vi "Top Level FPGA_w8LED.vi"() -> ()   [LabVIEW 2012]
uses:
  <vilib>/Platform/TimedLoop/XDataNode/timing_clust.ctl
  <vilib>/Platform/TimedLoop/XDataNode/nitl_modes.ctl
  <vilib>/Platform/TimedLoop/XDataNode/wakeup.ctl
  <vilib>/rvi/DataTransferAndStorage/Container/Common/niFpgaContainerMetaDataKey.ctl
  <vilib>/rvi/DataTransferAndStorage/Container/Common/niFpgaContainerState.ctl
  <vilib>/rvi/DataTransferAndStorage/Container/Common/niFpgaDataTypeControl.ctl
  <vilib>/rvi/DataTransferAndStorage/Container/Common/niFpgaContainerImplementationControl.ctl
  <vilib>/rvi/DataTransferAndStorage/Container/Common/niFpgaContainerArbitrationOptionsControl.ctl
  <vilib>/rvi/DataTransferAndStorage/Container/Common/niFpgaTransferTypeControl.ctl
  <vilib>/rvi/DataTransferAndStorage/Container/Common/niFpgaContainerInitializationParameters.ctl
  <vilib>/rvi/Memory/Memory_Types/niFpgaMemoryInterfaceConfiguration.ctl
  <vilib>/rvi/FIFO/Fifo_Types/niFpgaFifoControlLogicControl.ctl
  <vilib>/rvi/eio/common/nirviEmuTemplateMethod_errors.vi
  <vilib>/rvi/FIFO/Fifo_Resource/nirvififoEmulationSetSize.vi
  <vilib>/rvi/DataTransferAndStorage/Container/Common/niFpgaContainerGetUniqueNameForEmu.vi
  <vilib>/rvi/Emulation/niFpgaSctlEmulationRegisterWithScheduler.vi
  <vilib>/rvi/Emulation/niFpgaSctlEmulationScheduler.vi
  <vilib>/rvi/DataTransferAndStorage/Container/Common/niFpgaContainerSetEmuInfo.vi
  <vilib>/rvi/eio/common/nirviEmuReportErrorAndStop.vi
  <vilib>/rvi/Emulation/niFpgaSctlEmulationFifoFullMgr.vi
  <vilib>/rvi/errors/niFpgaSetErrorForExecOnDevCompSimple.vi
  <vilib>/rvi/Memory/Memory_Emulation/nirvimemoryEmulationManagerCache_GetValue.vi
  <vilib>/rvi/Memory/Memory_Emulation/niFpgaMemoryEmulationValidateCache.vi
  <vilib>/rvi/Memory/Memory_Emulation/nirvimemoryEmulationManagerCache_InsertValue.vi
  <vilib>/rvi/Memory/Memory_Emulation/nirvimemoryEmulationManagerCache_SetValue.vi
  <vilib>/rvi/Emulation/niFpgaSctlEmulationResourceMgr.vi
  <vilib>/rvi/Memory/Memory_Emulation/niFpgaMemoryEmulationCacheClearOnFirstRun.vi
  <vilib>/rvi/Memory/Memory_Emulation/nirvimemoryEmulationManagerCache_MakeExclusive.vi
  <vilib>/rvi/Memory/Memory_Emulation/nirvimemoryEmulationManagerCache_ReleaseExclusive.vi
  <vilib>/Utility/error.llb/Clear Errors.vi
  <vilib>/eio/EIONode/EIONode.xnode
  <vilib>/Platform/TimedLoop/XDataNode/XDataNode.xnode
  <vilib>/rvi/DataTransferAndStorage/Container/XNode/niFpgaContainer.xnode
  <vilib>/rvi/FIFO/Fifo_Resource/nirvififoEmulationClear.vi
  <vilib>/rvi/LocalResourceManager/LocalResourceManager.xnode
  <vilib>/rvi/FIFO/Fifo_Resource/nirvififoEmulationRead.vi
  <vilib>/rvi/DataTransferAndStorage/Register/Emulation/niFpgaRegisterEmulation.vi
  <vilib>/rvi/Memory/Memory_Emulation/nirvimemoryEmulation.vi
  <vilib>/rvi/FIFO/Fifo_Resource/nirvififoEmulationWrite.vi
  <vilib>/Platform/TimedLoop/XDataNode/XDNodeRunTimeDep.lvlib
panel:
  in  "Testpulse separation (20 ns ticks)":u32=50000
  in  "channel 7 on/off":bool
  in  "channel 6 on/off":bool
  in  "channel 5 on/off":bool
  in  "channel 4 on/off":bool
  in  "channel 3 on/off":bool
  in  "channel 1 on/off":bool
  in  "channel 2 on/off":bool
  in  "channel 0 on/off":bool
  out "Timestamp":u64
  in  "Stop FPGA and exit":bool
  out "DMA FIFO Timed Out?":bool
  in  "Testpulser On/Off":bool
  in  "Testpulse Time Delay (20 ns ticks)":u32=15
  in  "Testpulse duration (20 ns ticks)":u32=1
  in  "location":i16(ring) items=["Purdue", "NIKHEF", "Zurich", "???"]
  in  "initial value":u64
  in  "circular buffer length":u32=1000
  in  "# of pretrigger":u32=20
  out "IO Module\\Pll Unlocked":bool
  out "IO Module\\ADC Error B":bool
  out "IO Module\\ADC Error A":bool
  out "Init Done":bool
  in  "Trigger 4":i16=4000
  in  "Trigger 5":i16=4000
  in  "Trigger 6":i16=4000
  in  "Trigger 7":i16=4000
  in  "Trigger 2":i16=4000
  in  "Trigger 3":i16=4000
  in  "Trigger 1":i16=4000
  in  "Record Size only data":u32=95
  in  "Trigger 0":i16=4000
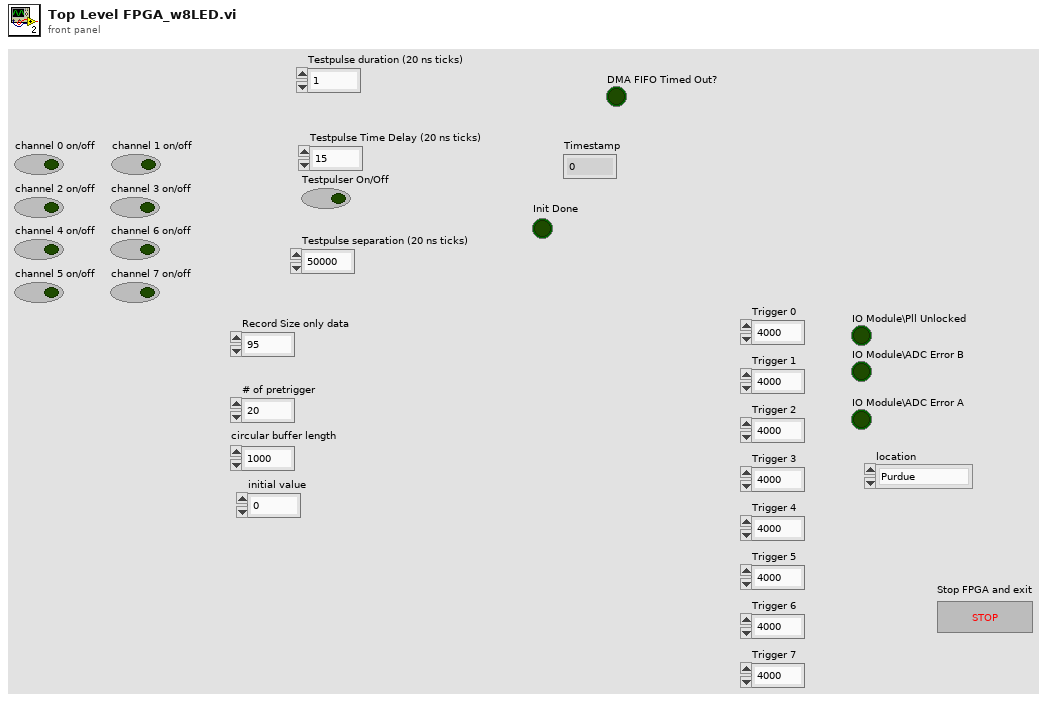
[diagram p1: front panel]
types:
  T1 = typedef "XDNodeRunTimeDep.lvlib/timing_clust.ctl" = cluster{"Expected End [f-1]":u64, "Actual End [f-1]":u64, "Finished Late? [f-1]":bool, "Expected End [i-1]":u64, "Actual End [i-1]":u64, "Finished Late? [i-1]":bool, "Expected Start [i]":u64, "Actual Start [i]":u64, "Expected Start [f]":u64, "Actual Start [f]":u64, "Source Name":string, "Structure Name":string, "Period":i64, "Deadline":i64, "Offset":i64, "Start":i64, "Priority":i32, "Timeout":i32, "Mode":T2, "Wakeup Reason":T3, "Error":errorcluster, "Source Type":string, "Secondary Source Type":string, "Global End Time":u64, "Global Start Time":u64, "Frame Duration":u64, "Iteration Duration":u64, "Assigned CPU":i32, "I/O Scan Engine Mode":u32}
  T2 = typedef "XDNodeRunTimeDep.lvlib/nitl_modes.ctl" = enum32{"No Change", "Process missed periods, maintain original phase", "Discard missed periods, maintain original phase", "Process missed periods, ignore original phase", "Discard missed periods, ignore original phase"}
  T3 = typedef "XDNodeRunTimeDep.lvlib/wakeup.ctl" = enum32{"Normal", "Aborted", "Asynchronous wakeup", "Timing source error", "Timed loop error", "Timeout"}
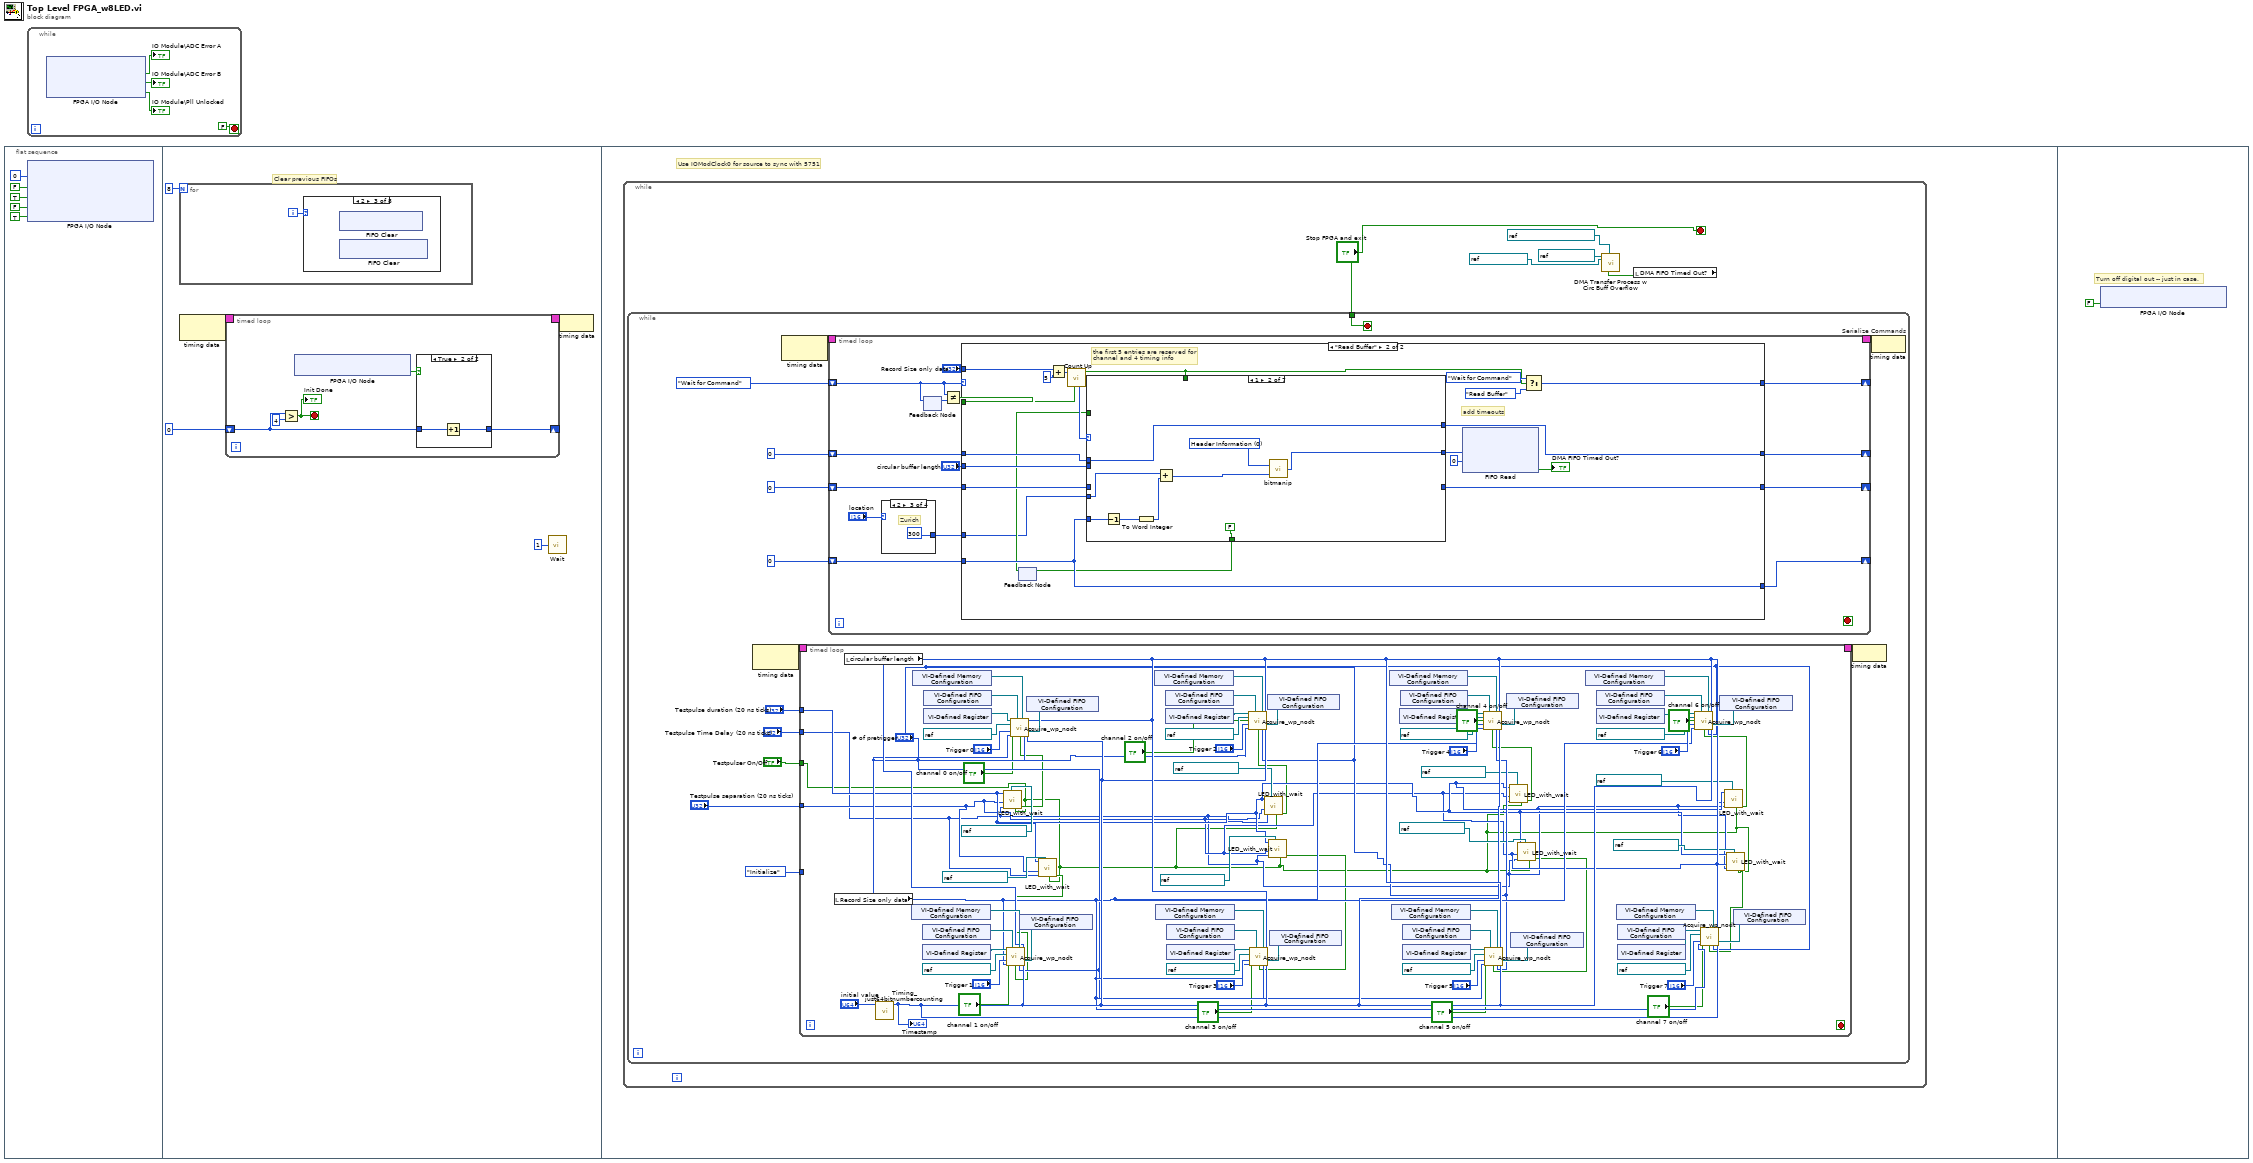
[diagram p0: block diagram]
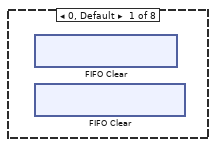
[diagram p2: hidden frame]
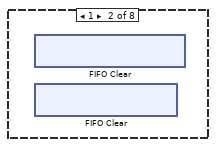
[diagram p3: hidden frame]
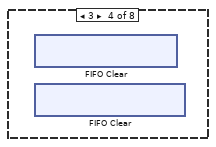
[diagram p4: hidden frame]
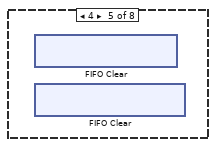
[diagram p5: hidden frame]
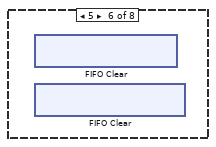
[diagram p6: hidden frame]
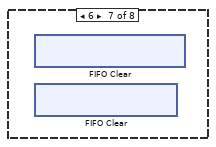
[diagram p7: hidden frame]
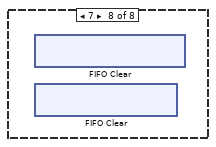
[diagram p8: hidden frame]
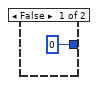
[diagram p9: hidden frame]
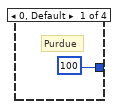
[diagram p10: hidden frame]
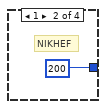
[diagram p11: hidden frame]
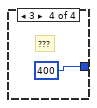
[diagram p12: hidden frame]
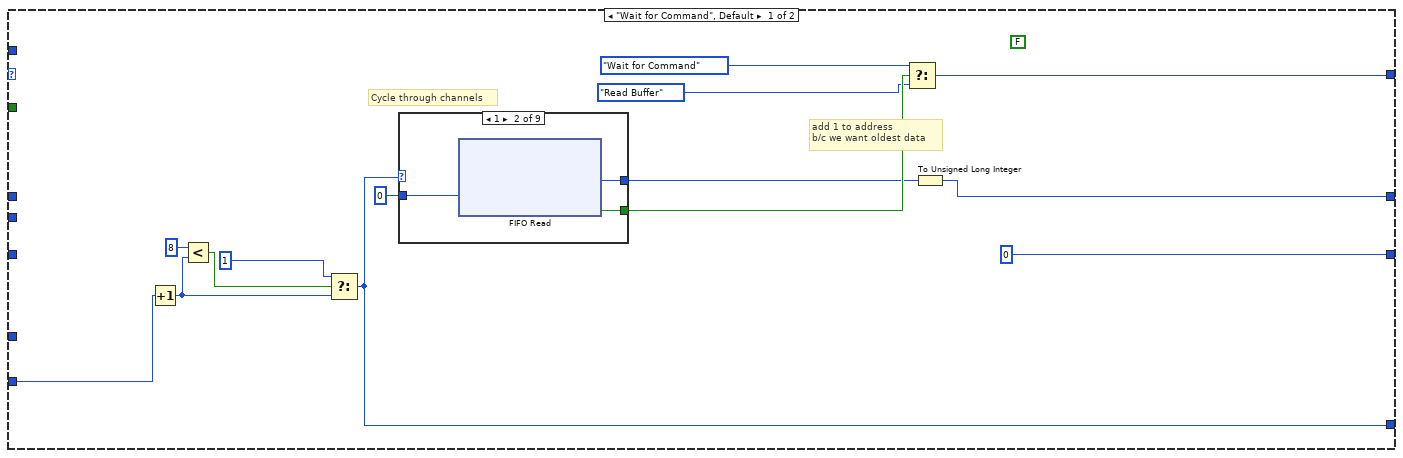
[diagram p13: hidden frame]
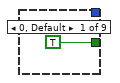
[diagram p14: hidden frame]
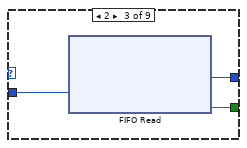
[diagram p15: hidden frame]
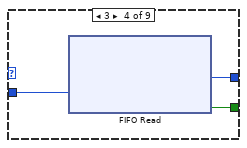
[diagram p16: hidden frame]
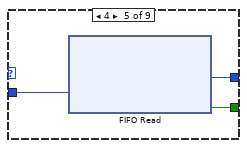
[diagram p17: hidden frame]
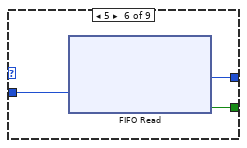
[diagram p18: hidden frame]
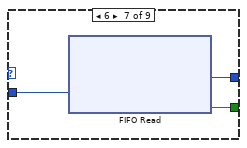
[diagram p19: hidden frame]
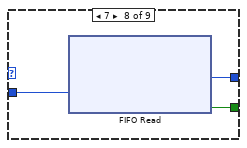
[diagram p20: hidden frame]
diagram:
  n1 = flat-sequence {
    frame #0 {
      n2 = xnode "FPGA I/O Node"("IO Module\\Sample Clock Select"=u8 0 ("IO Module\\Sample Clock Select"), "IO Module\\Force Initialization"=FALSE ("IO Module\\Force Initialization"), "IO Module\\Force Initialization"=TRUE ("IO Module\\Force Initialization"), "IO Module\\Force Initialization"=FALSE ("IO Module\\Force Initialization"), "IO Module\\Digital Output Enable"=TRUE ("IO Module\\Digital Output Enable")) -> ()  [unwired: 5 in, 5 out]
    }
    frame #1 {
      # "Clear previous FIFOs"
      n3 = for {
        N: 8 -> [_]
        i -> [w11]
        n4 = case shown="2" w11 {
          frame 0, Default {
            n5 = xnode ("FIFO Clear")() -> ()  [unwired: 1 in, 1 out]
            n6 = xnode ("FIFO Clear")() -> ()  [unwired: 1 in, 1 out]
          }
          frame 1 {
            n7 = xnode ("FIFO Clear")() -> ()  [unwired: 1 in, 1 out]
            n8 = xnode ("FIFO Clear")() -> ()  [unwired: 1 in, 1 out]
          }
          frame 2 {
            n9 = xnode ("FIFO Clear")() -> ()  [unwired: 1 in, 1 out]
            n10 = xnode ("FIFO Clear")() -> ()  [unwired: 1 in, 1 out]
          }
          frame 3 {
            n11 = xnode ("FIFO Clear")() -> ()  [unwired: 1 in, 1 out]
            n12 = xnode ("FIFO Clear")() -> ()  [unwired: 1 in, 1 out]
          }
          frame 4 {
            n13 = xnode ("FIFO Clear")() -> ()  [unwired: 1 in, 1 out]
            n14 = xnode ("FIFO Clear")() -> ()  [unwired: 1 in, 1 out]
          }
          frame 5 {
            n15 = xnode ("FIFO Clear")() -> ()  [unwired: 1 in, 1 out]
            n16 = xnode ("FIFO Clear")() -> ()  [unwired: 1 in, 1 out]
          }
          frame 6 {
            n17 = xnode ("FIFO Clear")() -> ()  [unwired: 1 in, 1 out]
            n18 = xnode ("FIFO Clear")() -> ()  [unwired: 1 in, 1 out]
          }
          frame 7 {
            n19 = xnode ("FIFO Clear")() -> ()  [unwired: 1 in, 1 out]
            n20 = xnode ("FIFO Clear")() -> ()  [unwired: 1 in, 1 out]
          }
        }
      }
      n21 = node-c288() -> (w10:T1)  [unwired: 1 in]
      n22 = timed-loop {
        shift-right: [w15] -> _
        shift-left: u16 0 -> [w14]
        timing: w10 -> [_]
        timing-out: [_] -> w9
        stop <- w12 stop-if-true
        n23 = Greater?(x=w14, y=u16 4) -> (0:w12:bool)
        "Init Done" <- w12
        n24 = xnode "FPGA I/O Node"() -> ("IO Module\\Initialization Done"=w16:bool)  [unwired: 1 in, 1 out]
        n25 = case shown="True" w16 {
          tunnel: [u16 0 w19] -> w15
          tunnel: w14 -> [_ w18]
          frame False {
          }
          frame True {
            n26 = Increment(x=w18) -> (x+1=w19:u16)
          }
        }
      }
      n27 = call "Wait"("Count(mSec)"=u32 1) -> ()  [unwired: 1 out]
      n28 = node-c288(w9) -> ()
    }
    frame #2 {
      # "Use IOModClock0 for source to sync with 5751"
      n29 = while {
        stop <- "Stop FPGA and exit" stop-if-true
        n30 = while {
          tunnel: "Stop FPGA and exit" -> [w34]
          stop <- w34 stop-if-true
          n31 = node-c288() -> (w40:T1)  [unwired: 1 in]
          n32 = node-c288() -> (w42:T1)  [unwired: 1 in]
          n33 = timed-loop {
            timing: w40 -> [_]
            timing-out: [_] -> w39
            tunnel: "Testpulser On/Off" -> [w43]
            tunnel: "Testpulse Time Delay (20 ns ticks)" -> [w50]
            tunnel: "Testpulse duration (20 ns ticks)" -> [w52]
            tunnel: enum16{"Initialize", "Get New Value", "Wait"}."Initialize" ("State In") -> [_]
            tunnel: "Testpulse separation (20 ns ticks)" -> [w51]
            stop <- _ stop-if-true
            n34 = local read "Record Size only data"() -> (w73:u32)
            n35 = local read "circular buffer length"() -> (w75:u32)
            n36 = call "Timing_just64bitnumbercounting.vi"("initial value"="initial value") -> ("x+1"=w74:u64)  [unwired: 10 in]
            "Timestamp" <- w74
            n37 = xnode "VI-Defined Memory Configuration"() -> ("Memory Out"=w122:refnum<k21>)
            n38 = xnode "VI-Defined Memory Configuration"() -> ("Memory Out"=w76:refnum<k21>)
            n39 = xnode "VI-Defined FIFO Configuration"() -> ("FIFO Out"=w121:refnum<k21>)
            n40 = xnode "VI-Defined Register"() -> ("Register Out"=w102:refnum<k21>)
            n41 = xnode "VI-Defined FIFO Configuration"() -> ("FIFO Out"=w77:refnum<k21>)
            n42 = xnode "VI-Defined Register"() -> ("Register Out"=w72:refnum<k21>)
            n43 = call "LED_with_wait.vi"("Testpulser On/Off"=w43, "FPGA I/O In"=refnum<k21> "IO Module\\D0 0", "Testpulse Time Delay (20 ns ticks)"=w50, "Testpulse Separation (20 ns ticks)"=w51, "Testpulse duration (20 ns ticks)"=w52) -> ("Is Test Pulse?"=w61:bool)  [unwired: 5 in, 1 out]
            n44 = xnode "VI-Defined FIFO Configuration"() -> ("FIFO Out"=w88:refnum<k21>)
            n45 = xnode "VI-Defined FIFO Configuration"() -> ("FIFO Out"=w80:refnum<k21>)
            n46 = call "Acquire_wp_nodt.vi"("Ch Armed Reg"=w72, "Command FIFO"=w77, "Circular Buffer Mem"=w76, "circular buffer length"=w75, "FPGA I/O In"=refnum<k21> "IO Module\\AI A0", "channel on/off"="channel 0 on/off", "Trigger"="Trigger 0", "Timing FIFO"=w80, "Samples to Acquire"=w73, "Is Test Pulse?"=w61, "# of pretrigger"="# of pretrigger", "timing"=w74) -> ()  [unwired: 4 in]
            n47 = call "LED_with_wait.vi"("Testpulser On/Off"=w43, "FPGA I/O In"=refnum<k21> "IO Module\\D0 1", "Testpulse Time Delay (20 ns ticks)"=w50, "Testpulse Separation (20 ns ticks)"=w51, "Testpulse duration (20 ns ticks)"=w52) -> ("Is Test Pulse?"=w60:bool)  [unwired: 5 in, 1 out]
            n48 = call "Acquire_wp_nodt.vi"("Ch Armed Reg"=w102, "Command FIFO"=w121, "Circular Buffer Mem"=w122, "circular buffer length"=w75, "FPGA I/O In"=refnum<k21> "IO Module\\AI A1", "channel on/off"="channel 1 on/off", "Trigger"="Trigger 1", "Timing FIFO"=w88, "Samples to Acquire"=w73, "Is Test Pulse?"=w60, "# of pretrigger"="# of pretrigger", "timing"=w74) -> ()  [unwired: 4 in]
            n49 = xnode "VI-Defined Memory Configuration"() -> ("Memory Out"=w116:refnum<k21>)
            n50 = xnode "VI-Defined Memory Configuration"() -> ("Memory Out"=w119:refnum<k21>)
            n51 = xnode "VI-Defined FIFO Configuration"() -> ("FIFO Out"=w115:refnum<k21>)
            n52 = xnode "VI-Defined Register"() -> ("Register Out"=w98:refnum<k21>)
            n53 = xnode "VI-Defined FIFO Configuration"() -> ("FIFO Out"=w120:refnum<k21>)
            n54 = xnode "VI-Defined Register"() -> ("Register Out"=w100:refnum<k21>)
            n55 = call "LED_with_wait.vi"("Testpulser On/Off"=w43, "FPGA I/O In"=refnum<k21> "IO Module\\D0 2", "Testpulse Time Delay (20 ns ticks)"=w50, "Testpulse Separation (20 ns ticks)"=w51, "Testpulse duration (20 ns ticks)"=w52) -> ("Is Test Pulse?"=w45:bool)  [unwired: 5 in, 1 out]
            n56 = xnode "VI-Defined FIFO Configuration"() -> ("FIFO Out"=w87:refnum<k21>)
            n57 = call "Acquire_wp_nodt.vi"("Ch Armed Reg"=w98, "Command FIFO"=w115, "Circular Buffer Mem"=w116, "circular buffer length"=w75, "FPGA I/O In"=refnum<k21> "IO Module\\AI A2", "channel on/off"="channel 2 on/off", "Trigger"="Trigger 2", "Timing FIFO"=w87, "Samples to Acquire"=w73, "Is Test Pulse?"=w45, "# of pretrigger"="# of pretrigger", "timing"=w74) -> ()  [unwired: 4 in]
            n58 = call "LED_with_wait.vi"("Testpulser On/Off"=w43, "FPGA I/O In"=refnum<k21> "IO Module\\D0 3", "Testpulse Time Delay (20 ns ticks)"=w50, "Testpulse Separation (20 ns ticks)"=w51, "Testpulse duration (20 ns ticks)"=w52) -> ("Is Test Pulse?"=w44:bool)  [unwired: 5 in, 1 out]
            n59 = xnode "VI-Defined FIFO Configuration"() -> ("FIFO Out"=w86:refnum<k21>)
            n60 = call "Acquire_wp_nodt.vi"("Ch Armed Reg"=w100, "Command FIFO"=w120, "Circular Buffer Mem"=w119, "circular buffer length"=w75, "FPGA I/O In"=refnum<k21> "IO Module\\AI A3", "channel on/off"="channel 3 on/off", "Trigger"="Trigger 3", "Timing FIFO"=w86, "Samples to Acquire"=w73, "Is Test Pulse?"=w44, "# of pretrigger"="# of pretrigger", "timing"=w74) -> ()  [unwired: 4 in]
            n61 = xnode "VI-Defined Memory Configuration"() -> ("Memory Out"=w104:refnum<k21>)
            n62 = xnode "VI-Defined Memory Configuration"() -> ("Memory Out"=w107:refnum<k21>)
            n63 = xnode "VI-Defined Register"() -> ("Register Out"=w92:refnum<k21>)
            n64 = xnode "VI-Defined FIFO Configuration"() -> ("FIFO Out"=w103:refnum<k21>)
            n65 = xnode "VI-Defined FIFO Configuration"() -> ("FIFO Out"=w108:refnum<k21>)
            n66 = xnode "VI-Defined Register"() -> ("Register Out"=w96:refnum<k21>)
            n67 = xnode "VI-Defined FIFO Configuration"() -> ("FIFO Out"=w85:refnum<k21>)
            n68 = call "LED_with_wait.vi"("Testpulser On/Off"=w43, "FPGA I/O In"=refnum<k21> "IO Module\\D0 4", "Testpulse Time Delay (20 ns ticks)"=w50, "Testpulse Separation (20 ns ticks)"=w51, "Testpulse duration (20 ns ticks)"=w52) -> ("Is Test Pulse?"=w46:bool)  [unwired: 5 in, 1 out]
            n69 = call "Acquire_wp_nodt.vi"("Ch Armed Reg"=w92, "Command FIFO"=w103, "Circular Buffer Mem"=w104, "circular buffer length"=w75, "FPGA I/O In"=refnum<k21> "IO Module\\AI A4", "channel on/off"="channel 4 on/off", "Trigger"="Trigger 4", "Timing FIFO"=w85, "Samples to Acquire"=w73, "Is Test Pulse?"=w46, "# of pretrigger"="# of pretrigger", "timing"=w74) -> ()  [unwired: 4 in]
            n70 = xnode "VI-Defined FIFO Configuration"() -> ("FIFO Out"=w84:refnum<k21>)
            n71 = call "LED_with_wait.vi"("Testpulser On/Off"=w43, "FPGA I/O In"=refnum<k21> "IO Module\\D0 5", "Testpulse Time Delay (20 ns ticks)"=w50, "Testpulse Separation (20 ns ticks)"=w51, "Testpulse duration (20 ns ticks)"=w52) -> ("Is Test Pulse?"=w47:bool)  [unwired: 5 in, 1 out]
            n72 = call "Acquire_wp_nodt.vi"("Ch Armed Reg"=w96, "Command FIFO"=w108, "Circular Buffer Mem"=w107, "circular buffer length"=w75, "FPGA I/O In"=refnum<k21> "IO Module\\AI A5", "channel on/off"="channel 5 on/off", "Trigger"="Trigger 5", "Timing FIFO"=w84, "Samples to Acquire"=w73, "Is Test Pulse?"=w47, "# of pretrigger"="# of pretrigger", "timing"=w74) -> ()  [unwired: 4 in]
            n73 = xnode "VI-Defined Memory Configuration"() -> ("Memory Out"=w113:refnum<k21>)
            n74 = xnode "VI-Defined FIFO Configuration"() -> ("FIFO Out"=w114:refnum<k21>)
            n75 = xnode "VI-Defined Register"() -> ("Register Out"=w94:refnum<k21>)
            n76 = xnode "VI-Defined Memory Configuration"() -> ("Memory Out"=w110:refnum<k21>)
            n77 = xnode "VI-Defined FIFO Configuration"() -> ("FIFO Out"=w109:refnum<k21>)
            n78 = xnode "VI-Defined Register"() -> ("Register Out"=w90:refnum<k21>)
            n79 = xnode "VI-Defined FIFO Configuration"() -> ("FIFO Out"=w83:refnum<k21>)
            n80 = call "LED_with_wait.vi"("Testpulser On/Off"=w43, "FPGA I/O In"=refnum<k21> "IO Module\\D0 6", "Testpulse Time Delay (20 ns ticks)"=w50, "Testpulse Separation (20 ns ticks)"=w51, "Testpulse duration (20 ns ticks)"=w52) -> ("Is Test Pulse?"=w48:bool)  [unwired: 5 in, 1 out]
            n81 = call "Acquire_wp_nodt.vi"("Ch Armed Reg"=w94, "Command FIFO"=w114, "Circular Buffer Mem"=w113, "circular buffer length"=w75, "FPGA I/O In"=refnum<k21> "IO Module\\AI A6", "channel on/off"="channel 6 on/off", "Trigger"="Trigger 6", "Timing FIFO"=w83, "Samples to Acquire"=w73, "Is Test Pulse?"=w48, "# of pretrigger"="# of pretrigger", "timing"=w74) -> ()  [unwired: 4 in]
            n82 = call "LED_with_wait.vi"("Testpulser On/Off"=w43, "FPGA I/O In"=refnum<k21> "IO Module\\D0 7", "Testpulse Time Delay (20 ns ticks)"=w50, "Testpulse Separation (20 ns ticks)"=w51, "Testpulse duration (20 ns ticks)"=w52) -> ("Is Test Pulse?"=w49:bool)  [unwired: 5 in, 1 out]
            n83 = xnode "VI-Defined FIFO Configuration"() -> ("FIFO Out"=w82:refnum<k21>)
            n84 = call "Acquire_wp_nodt.vi"("Ch Armed Reg"=w90, "Command FIFO"=w109, "Circular Buffer Mem"=w110, "circular buffer length"=w75, "FPGA I/O In"=refnum<k21> "IO Module\\AI A7", "channel on/off"="channel 7 on/off", "Trigger"="Trigger 7", "Timing FIFO"=w82, "Samples to Acquire"=w73, "Is Test Pulse?"=w49, "# of pretrigger"="# of pretrigger", "timing"=w74) -> ()  [unwired: 4 in]
          }
          n85 = timed-loop "Serialize Commands" {
            timing: w42 -> [_]
            timing-out: [_] -> w41
            shift-right: [w904] -> _
            shift-left: enum16{"Wait for Command", "Read Buffer"}."Wait for Command" -> [w902]
            shift-right: [w908] -> _
            shift-left: u32 0 ("Element") -> [w907]
            shift-right: [w906] -> _
            shift-left: u8 0 ("t") -> [w905]
            shift-right: [w899] -> _
            shift-left: u64 0 ("Element") -> [w898]
            stop <- _ stop-if-true
            n86 = case shown="2" "location" {
              tunnel: [i16 100 i16 200 i16 300 i16 400] -> w896
              frame 0, Default {
                # "Purdue"
              }
              frame 1 {
                # "NIKHEF"
              }
              frame 2 {
                # "Zurich"
              }
              frame 3 {
                # "???"
              }
            }
            n87 = feedback-in #1(w902) -> ()
            n88 = feedback #1() -> (w903:enum16{"Wait for Command", "Read Buffer"})  [unwired: 1 in]
            n89 = Not Equal?(x=w902, y=w903) -> (x != y?=w900:bool)
            n90 = case shown="\"Read Buffer\"" w902 {
              tunnel: "Record Size only data" -> [_ w962]
              tunnel: [w916 w972] -> w906
              tunnel: w905 -> [w918 w972]
              tunnel: [w919 w957] -> w908
              tunnel: w907 -> [_ w971]
              tunnel: [w922 w973] -> w904
              tunnel: "circular buffer length" -> [_ w970]
              tunnel: w900 -> [_ w964]
              tunnel: [u64 0 ("Element") w959] -> w899
              tunnel: w898 -> [_ w958]
              tunnel: w896 -> [_ w953]
              frame "Wait for Command", Default {
                (unwired) FALSE
                # "add 1 to address\nb/c we want oldest data"
                # "Cycle through channels"
                n91 = Increment(x=w918) -> (x+1=w917:u8)
                n92 = Less?(x=u8 8, y=w917) -> (x < y?=w926:bool)
                n93 = Select(t=u8 1, s=w926, f=w917) -> (s? t:f=w916:u8)
                n94 = case shown="1" w916 {
                  tunnel: [TRUE ("Timed Out?") w931 w932 w935 w938 w941 w944 w947 w950] -> w923
                  tunnel: 0 ("Timeout") -> [_ w930 w934 w937 w940 w943 w946 w949 w952]
                  tunnel: [_ w929 w933 w936 w939 w942 w945 w948 w951] -> w915
                  frame 0, Default {
                  }
                  frame 1 {
                    n95 = xnode ("FIFO Read")("Timeout"=w930) -> ("Element"=w929:i16, "Timed Out?"=w931:bool)  [unwired: 1 in, 1 out]
                  }
                  frame 2 {
                    n96 = xnode ("FIFO Read")("Timeout"=w934) -> ("Element"=w933:i16, "Timed Out?"=w932:bool)  [unwired: 1 in, 1 out]
                  }
                  frame 3 {
                    n97 = xnode ("FIFO Read")("Timeout"=w937) -> ("Element"=w936:i16, "Timed Out?"=w935:bool)  [unwired: 1 in, 1 out]
                  }
                  frame 4 {
                    n98 = xnode ("FIFO Read")("Timeout"=w940) -> ("Element"=w939:i16, "Timed Out?"=w938:bool)  [unwired: 1 in, 1 out]
                  }
                  frame 5 {
                    n99 = xnode ("FIFO Read")("Timeout"=w943) -> ("Element"=w942:i16, "Timed Out?"=w941:bool)  [unwired: 1 in, 1 out]
                  }
                  frame 6 {
                    n100 = xnode ("FIFO Read")("Timeout"=w946) -> ("Element"=w945:i16, "Timed Out?"=w944:bool)  [unwired: 1 in, 1 out]
                  }
                  frame 7 {
                    n101 = xnode ("FIFO Read")("Timeout"=w949) -> ("Element"=w948:i16, "Timed Out?"=w947:bool)  [unwired: 1 in, 1 out]
                  }
                  frame 8 {
                    n102 = xnode ("FIFO Read")("Timeout"=w952) -> ("Element"=w951:i16, "Timed Out?"=w950:bool)  [unwired: 1 in, 1 out]
                  }
                }
                n103 = Select(t=enum16{"Wait for Command", "Read Buffer"}."Wait for Command", s=w923, f=enum16{"Wait for Command", "Read Buffer"}."Read Buffer") -> (s? t:f=w922:enum16{"Wait for Command", "Read Buffer"})
                n104 = To Unsigned Long Integer(number=w915) -> (unsigned 32bit integer=w919:u32)
              }
              frame "Read Buffer" {
                # "the first 5 entries are reserved for channel and 4 timing info"
                # "add timeouts"
                n105 = feedback #2() -> (w956:bool)  [unwired: 1 in]
                n106 = Add(x=w962, y=u32 5) -> (x+y=w960:u32)
                n107 = call "Count Up.vi"("Reset?"=w964, "goal"=w960) -> ("Count Met"=w966:bool, "count"=w963:u32)  [unwired: 8 in]
                n108 = case shown="1" w963 {
                  tunnel: w972 -> [_ w980 w989 _ _ _ w1028]
                  tunnel: w971 -> [_ w986 w991 w1012 w1018 w1024 w1035]
                  tunnel: w970 -> [_ _ _ _ _ _ w1034]
                  tunnel: w966 -> [_ _ _ _ _ _ w1033]
                  tunnel: [i16 0 ("Data") w983 w993 w1010 w1016 w1022 w1029] -> w965
                  tunnel: w956 -> [_ _ _ _ _ _ w1031]
                  tunnel: [u64 0 ("Element") _ w990 w1013 w1019 w1025 _] -> w959
                  tunnel: w958 -> [_ _ _ w1013 w1019 w1025 _]
                  tunnel: [u32 0 ("Element") w986 w991 w1012 w1018 w1024 _] -> w957
                  tunnel: [FALSE FALSE FALSE FALSE FALSE TRUE FALSE] -> w955
                  tunnel: w953 -> [_ w978 _ _ _ _ _]
                  frame 0, Default {
                  }
                  frame 1 {
                    w982 = u16 0 items=["Header Information", "Particle Pulse", "Test Pulse"] ("Pulse Type")
                    n109 = Decrement(x=w980) -> (x-1=w981:u8)
                    n110 = To Word Integer(number=w981) -> (16bit integer=w979:i16)
                    n111 = Add(x=w978, y=w979) -> (x+y=w984:i16)
                    n112 = call "bitmanip.vi"("Pulse Type"=w982, "Integer to be written"=w984) -> ("Integer Written"=w983:i16)  [unwired: 2 in]
                  }
                  frame 2 {
                    # "reads out the lsb of the timing information"
                    n113 = case shown="2" w989 {
                      tunnel: [_ w994 w996 w998 w1000 w1002 w1004 w1006 w1008] -> w990
                      frame Default {
                      }
                      frame 1 {
                        n114 = xnode ("FIFO Read")("Timeout"=0) -> ("Element"=w994:u64)  [unwired: 1 in, 2 out]
                      }
                      frame 2 {
                        n115 = xnode ("FIFO Read")("Timeout"=0) -> ("Element"=w996:u64)  [unwired: 1 in, 2 out]
                      }
                      frame 3 {
                        n116 = xnode ("FIFO Read")("Timeout"=0) -> ("Element"=w998:u64)  [unwired: 1 in, 2 out]
                      }
                      frame 4 {
                        n117 = xnode ("FIFO Read")("Timeout"=0) -> ("Element"=w1000:u64)  [unwired: 1 in, 2 out]
                      }
                      frame 5 {
                        n118 = xnode ("FIFO Read")("Timeout"=0) -> ("Element"=w1002:u64)  [unwired: 1 in, 2 out]
                      }
                      frame 6 {
                        n119 = xnode ("FIFO Read")("Timeout"=0) -> ("Element"=w1004:u64)  [unwired: 1 in, 2 out]
                      }
                      frame 7 {
                        n120 = xnode ("FIFO Read")("Timeout"=0) -> ("Element"=w1006:u64)  [unwired: 1 in, 2 out]
                      }
                      frame 8 {
                        n121 = xnode ("FIFO Read")("Timeout"=0) -> ("Element"=w1008:u64)  [unwired: 1 in, 2 out]
                      }
                    }
                    n122 = Split Number(x=w990) -> (hi(x)=w988:u32)  [unwired: 1 out]
                    n123 = Split Number(x=w988) -> (hi(x)=w987:u16)  [unwired: 1 out]
                    n124 = To Word Integer(number=w987) -> (16bit integer=w993:i16)
                  }
                  frame 3 {
                    n125 = Split Number(x=w1013) -> (hi(x)=w1015:u32)  [unwired: 1 out]
                    n126 = Split Number(x=w1015) -> (lo(x)=w1014:u16)  [unwired: 1 out]
                    n127 = To Word Integer(number=w1014) -> (16bit integer=w1010:i16)
                  }
                  frame 4 {
                    n128 = Split Number(x=w1019) -> (lo(x)=w1021:u32)  [unwired: 1 out]
                    n129 = Split Number(x=w1021) -> (hi(x)=w1020:u16)  [unwired: 1 out]
                    n130 = To Word Integer(number=w1020) -> (16bit integer=w1016:i16)
                  }
                  frame 5 {
                    n131 = Split Number(x=w1025) -> (lo(x)=w1027:u32)  [unwired: 1 out]
                    n132 = Split Number(x=w1027) -> (lo(x)=w1026:u16)  [unwired: 1 out]
                    n133 = To Word Integer(number=w1026) -> (16bit integer=w1022:i16)
                  }
                  frame 6.. {
                    n134 = call "Circular Buffer Address_try_without_deadtime.vi"("Reset?"=w1031, "Starting Address"=w1035, "circular buffer length"=w1034) -> ("Address"=w1032:u32)  [unwired: 8 in]
                    n135 = case shown="1" w1028 {
                      tunnel: w1032 -> [_ w1039 w1042 w1045 w1048 w1051 w1054 w1057 w1060]
                      tunnel: w1033 -> [_ w1038 w1041 w1044 w1047 w1050 w1053 w1056 w1059]
                      tunnel: [i16 0 w1037 w1040 w1043 w1046 w1049 w1052 w1055 w1058] -> w1029
                      frame Default {
                        # "Error"
                      }
                      frame 1 {
                        n136 = xnode ("Memory Read")("Address"=w1039) -> ("Data"=w1037:i16)  [unwired: 1 in, 1 out]
                        n137 = xnode ("Register Write")("Data"=w1038) -> ()  [unwired: 1 in, 1 out]
                      }
                      frame 2 {
                        n138 = xnode ("Memory Read")("Address"=w1042) -> ("Data"=w1040:i16)  [unwired: 1 in, 1 out]
                        n139 = xnode ("Register Write")("Data"=w1041) -> ()  [unwired: 1 in, 1 out]
                      }
                      frame 3 {
                        n140 = xnode ("Memory Read")("Address"=w1045) -> ("Data"=w1043:i16)  [unwired: 1 in, 1 out]
                        n141 = xnode ("Register Write")("Data"=w1044) -> ()  [unwired: 1 in, 1 out]
                      }
                      frame 4 {
                        n142 = xnode ("Memory Read")("Address"=w1048) -> ("Data"=w1046:i16)  [unwired: 1 in, 1 out]
                        n143 = xnode ("Register Write")("Data"=w1047) -> ()  [unwired: 1 in, 1 out]
                      }
                      frame 5 {
                        n144 = xnode ("Memory Read")("Address"=w1051) -> ("Data"=w1049:i16)  [unwired: 1 in, 1 out]
                        n145 = xnode ("Register Write")("Data"=w1050) -> ()  [unwired: 1 in, 1 out]
                      }
                      frame 6 {
                        n146 = xnode ("Memory Read")("Address"=w1054) -> ("Data"=w1052:i16)  [unwired: 1 in, 1 out]
                        n147 = xnode ("Register Write")("Data"=w1053) -> ()  [unwired: 1 in, 1 out]
                      }
                      frame 7 {
                        n148 = xnode ("Memory Read")("Address"=w1057) -> ("Data"=w1055:i16)  [unwired: 1 in, 1 out]
                        n149 = xnode ("Register Write")("Data"=w1056) -> ()  [unwired: 1 in, 1 out]
                      }
                      frame 8 {
                        n150 = xnode ("Memory Read")("Address"=w1060) -> ("Data"=w1058:i16)  [unwired: 1 in, 1 out]
                        n151 = xnode ("Register Write")("Data"=w1059) -> ()  [unwired: 1 in, 1 out]
                      }
                    }
                  }
                }
                n152 = feedback-in #2(w955) -> ()
                n153 = xnode ("FIFO Read")("Element"=w965, "Timeout"=0) -> ("Timed Out?"=→"DMA FIFO Timed Out?":bool)  [unwired: 1 in, 1 out]
                n154 = Select(t=enum16{"Wait for Command", "Read Buffer"}."Wait for Command", s=w966, f=enum16{"Wait for Command", "Read Buffer"}."Read Buffer") -> (s? t:f=w973:enum16{"Wait for Command", "Read Buffer"})
              }
            }
          }
          n155 = node-c288(w39) -> ()
          n156 = node-c288(w41) -> ()
        }
        n157 = local read "DMA FIFO Timed Out?"() -> (w26:bool)
        n158 = call "DMA Transfer Process w Circ Buff Overflow.vi"("DMA Write Timed Out?"=w26, "Clock Domain"=refnum<k21> "40 MHz Onboard Clock", "Local"=refnum<k21> "To DMA FIFO", "DMA"=refnum<k21> "To Host FIFO") -> ()  [unwired: 8 in]
      }
    }
    frame #3 {
      # "Turn off digital out -- just in case."
      n159 = xnode "FPGA I/O Node"("IO Module\\Digital Output Enable"=FALSE ("IO Module\\Digital Output Enable")) -> ()  [unwired: 1 in, 1 out]
    }
  }
  n160 = while {
    stop <- FALSE stop-if-true
    n161 = xnode "FPGA I/O Node"() -> ("IO Module\\ADC Error A"=→"IO Module\\ADC Error A":bool, "IO Module\\ADC Error B"=→"IO Module\\ADC Error B":bool, "IO Module\\Pll Unlocked"=→"IO Module\\Pll Unlocked":bool)  [unwired: 3 in, 3 out]
  }
